vi "Clear Rfpm Switch Session.vi"(0 "Logical Name":string, 11 "error in (no error)":errorcluster) -> (15 "error out":errorcluster)   [LabVIEW 2023, in "RFFixtureCharact.RFPM.lvlib" / "RF Subsystem Session Provider.lvclass"]
uses:
  RF Subsystem Session Provider.lvclass
  Common/Data Cache/Type Definitions/Dictionary Operation.ctl
  Common/RFCalAndFixtureCharact.Common.lvlib
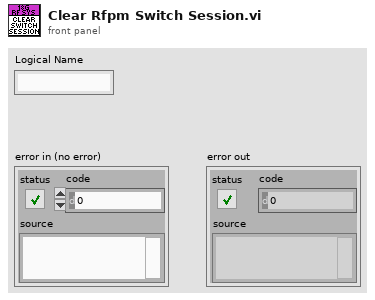
[diagram p1: front panel]
types:
  T1 = typedef "RFCalAndFixtureCharact.Common.lvlib/Dictionary Operation.ctl" = enum16{"Read", "Insert", "Remove", "Clear", "Get All", "Update"}
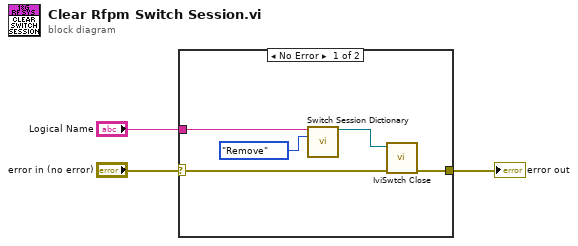
[diagram p0: block diagram]
diagram:
  n1 = case shown="No Error" "error in (no error)" {
    selector: "error in (no error)" -> [w8 w9]
    tunnel: [w7 w9] -> w2
    tunnel: "Logical Name" -> [w4 _]
    frame No Error {
      n2 = call "Switch Session Dictionary.vi"("Logical Name"=w4, "Action"=Dictionary_Operation."Remove") -> ("Ivi Switch Session Out"=w5:refnum<k15>)  [unwired: 11 in, 2 out]
      n3 = call <vilib>:"IviSwtch Close.vi"("error in (no error)"=w8, "instrument handle"=w5) -> ("error out"=w7:errorcluster)  [unwired: 9 in]
    }
    frame Error {
    }
  }
  "error out" <- w2
